vi "Verify New Data Type.vi"(5 "Selector":string, 7 "Menu":string, 8 "error in":errorcluster, 9 "Type Name":string, 10 "Type Directory":path) -> (0 "error out":errorcluster)   [LabVIEW 2020, in "Data Type Scripting.lvlib"]
doc: "_____\nCreated using DQMH Event Scripter 6.0.0.122."
uses:
  Data Type Scripting.lvlib
  Verify New Data Type Argument--cluster.ctl
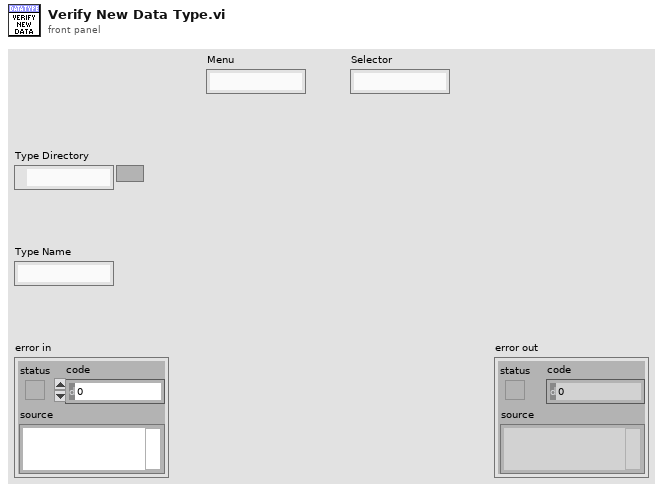
[diagram p1: front panel]
types:
  T1 = typedef "Data Type Scripting.lvlib/Verify New Data Type Argument--cluster.ctl" = cluster{"Type Directory":path, "Type Name":string, "Menu":string, "Selector":string}
  T2 = typedef "Data Type Scripting.lvlib/Request Events--cluster.ctl" = cluster{"Stop Module":refnum<user-event>, "Show Panel":refnum<user-event>, "Hide Panel":refnum<user-event>, "Get Module Execution Status":refnum<user-event>, "Show Diagram":refnum<user-event>, "Load Poly VI":refnum<user-event>, "Get Poly List":refnum<user-event>, "Get Poly Details":refnum<user-event>, "Open Poly VI Window":refnum<user-event>, "Create New Data Type":refnum<user-event>, "Verify New Data Type":refnum<user-event>}
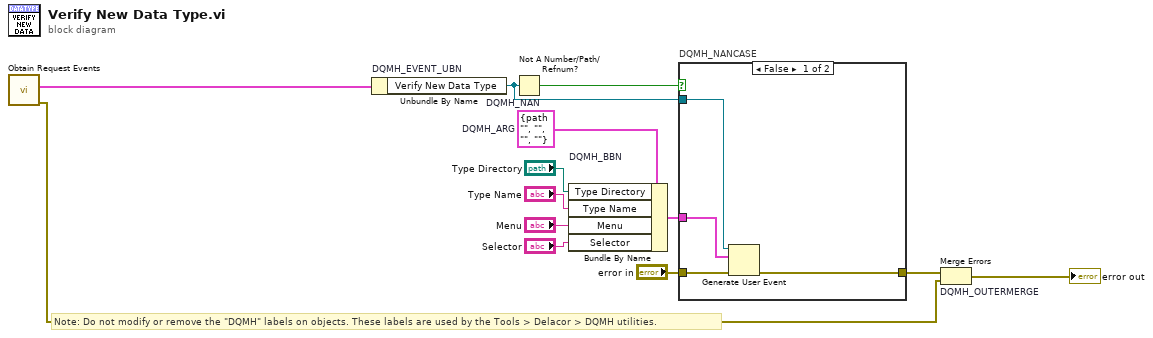
[diagram p0: block diagram]
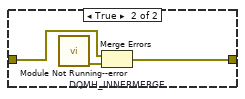
[diagram p2: hidden frame]
diagram:
  w7 = T1 {"Type Directory"=path "", "Type Name"="", "Menu"="", "Selector"=""}  # DQMH_ARG
  # "Note: Do not modify or remove the \"DQMH\" labels on objects. These labels are used by the Tools > Delacor > DQMH utilities."
  n1 = call "Obtain Request Events.vi"() -> ("error out"=w2:errorcluster, "Data Type Scripting Request Events"=w1:T2)  [unwired: 10 in]
  n2 = Unbundle By Name "DQMH_EVENT_UBN"(w1) -> ("Verify New Data Type"=w9:refnum<user-event>)
  n3 = Not A Number/Path/Refnum? "DQMH_NAN"(number/path/refnum=w9) -> (NaN/Path/Refnum?=w10:bool)
  n4 = Bundle By Name "DQMH_BBN"(cluster=w7, "Type Directory"="Type Directory", "Type Name"="Type Name", "Menu"="Menu", "Selector"="Selector") -> (w11:T1)
  n5 = case "DQMH_NANCASE" shown="False" w10 {
    tunnel: "error in" -> [w17 w20]
    tunnel: [w16 w19] -> w8
    tunnel: w9 -> [w15 _]
    tunnel: w11 -> [w14 _]
    frame False {
      n6 = Generate User Event(user event=w15, event data cluster=w14, error in=w17) -> (error out=w16:errorcluster)  [unwired: 1 in, 1 out]
    }
    frame True {
      n7 = call "Module Not Running--error.vi"() -> ("error out"=w18:errorcluster)  [unwired: 11 in]
      n8 = Merge Errors "DQMH_INNERMERGE"(w20, w18) -> (w19:errorcluster)
    }
  }
  n9 = Merge Errors "DQMH_OUTERMERGE"(w8, w2) -> (→"error out":errorcluster)
